vi "Actor Core.vi"(8 "error in":errorcluster, 11 "Bioreactor":refnum<class "Bioreactor.lvclass">) -> (0 "error out":errorcluster, 3 "Actor out":refnum<class "Actor.lvclass">)   [LabVIEW 2012, in "Bioreactor Actor.lvlib" / "Bioreactor.lvclass"]
doc: "This is Actor Core.vi, the main message handling loop for Actors. An actor usually just sits in this loop and processes messages as they arrive. Any error returned by the message Do.vi call will stop the loop, with error code 43 as the canonical signal to stop with no error sent to caller. Descendants may override that in Handle Error.vi."
uses:
  Bioreactor.lvclass
  <vilib>/ActorFramework/Actor/Actor.lvclass
  Bioreactor.lvclass/Bioreactor.ctl
  <vilib>/ActorFramework/Actor/Actor.lvclass/Actor.ctl
  <vilib>/ActorFramework/Message Enqueuer/Message Enqueuer.lvclass/Message Enqueuer.ctl
  <vilib>/ActorFramework/Message Enqueuer/Message Priority.ctl
  Read DVR.vi
  Write Loop Name.vi
  Write Graph History.vi
  Write Control Value.vi
  Write Control Graph.vi
  Write Process Setpoint.vi
  Write Process Value.vi
  Write Process Graph.vi
  Write VI Refnum.vi
  <vilib>/ActorFramework/Message Enqueuer/Init from Existing Queue.vi
  <vilib>/ActorFramework/Message Enqueuer/Enqueue.vi
  <vilib>/ActorFramework/Message Priority Queue/Priority Enqueue.vi
  <vilib>/ActorFramework/Message Enqueuer/Message Enqueuer.lvclass
  Bioreactor Messages/Read Setpoint Msg/Read Setpoint Msg.lvclass
  Bioreactor Messages/Read Output Msg/Read Output Msg.lvclass
  Bioreactor Messages/Read Value Msg/Read Value Msg.lvclass
  Bioreactor Messages/Update Indicators Msg/Update Indicators Msg.lvclass
  <vilib>/ActorFramework/Stop Msg/Stop Msg.lvclass
  Bioreactor Messages/Write Setpoint Msg/Write Setpoint Msg.lvclass
  Bioreactor Messages/Log Data Msg/Log Data Msg.lvclass
  Bioreactor Messages/Update Setpoint Msg/Update Setpoint Msg.lvclass
panel:
  in  "stop signal":bool
  out "Control Value":dbl=300.0
  in  "Graph History":dbl=300.0
  in  "Loop Name":u16(ring) caption="View"
  out "Control Graph":T1(graph) caption="Pump A"
  in  "Round Color Box 2":u32(colorbox)=16728642
  in  "Round Color Box":u32(colorbox)=483491
  in  "Process Setpoint":dbl=36.41913854673561
  out "Proccess Value":dbl=36.53012927910604
  out "Proccess Graph":T2(graph)
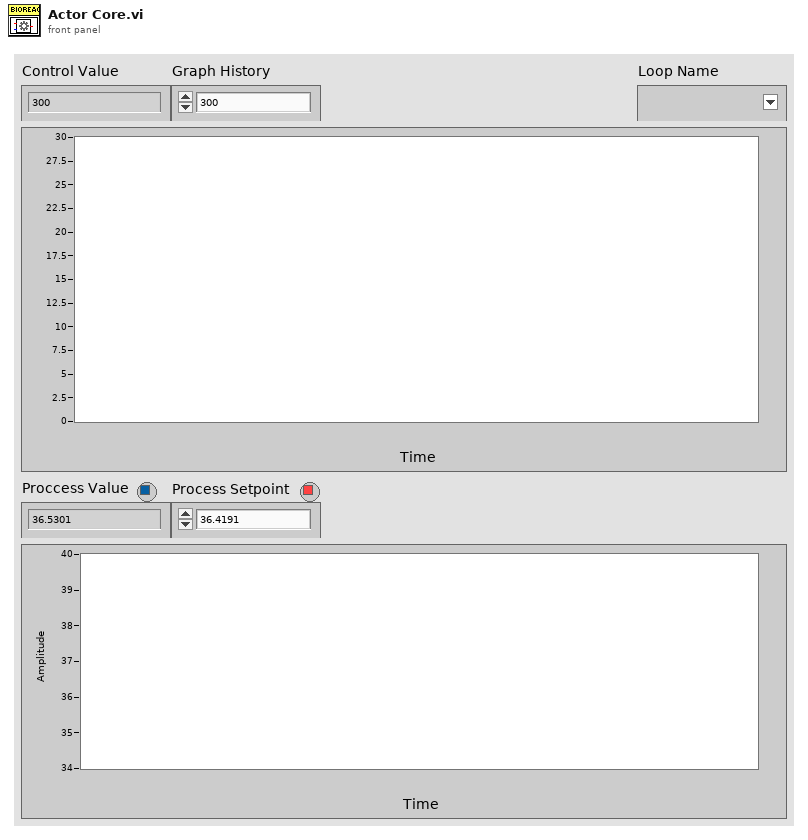
[diagram p1: front panel]
types:
  T1 = cluster{"output array":dbl[], "output array":dbl[]}
  T2 = cluster{"output array":dbl[], "output array":dbl[]}[]
  T3 = cluster{"Name":string, "Value":dbl, "Setpoint":dbl, "Output":dbl}[]
  T4 = typedef "Actor Framework.lvlib/Message Enqueuer.lvclass/Message Priority.ctl" = enum16{"Low", "Normal", "High"}
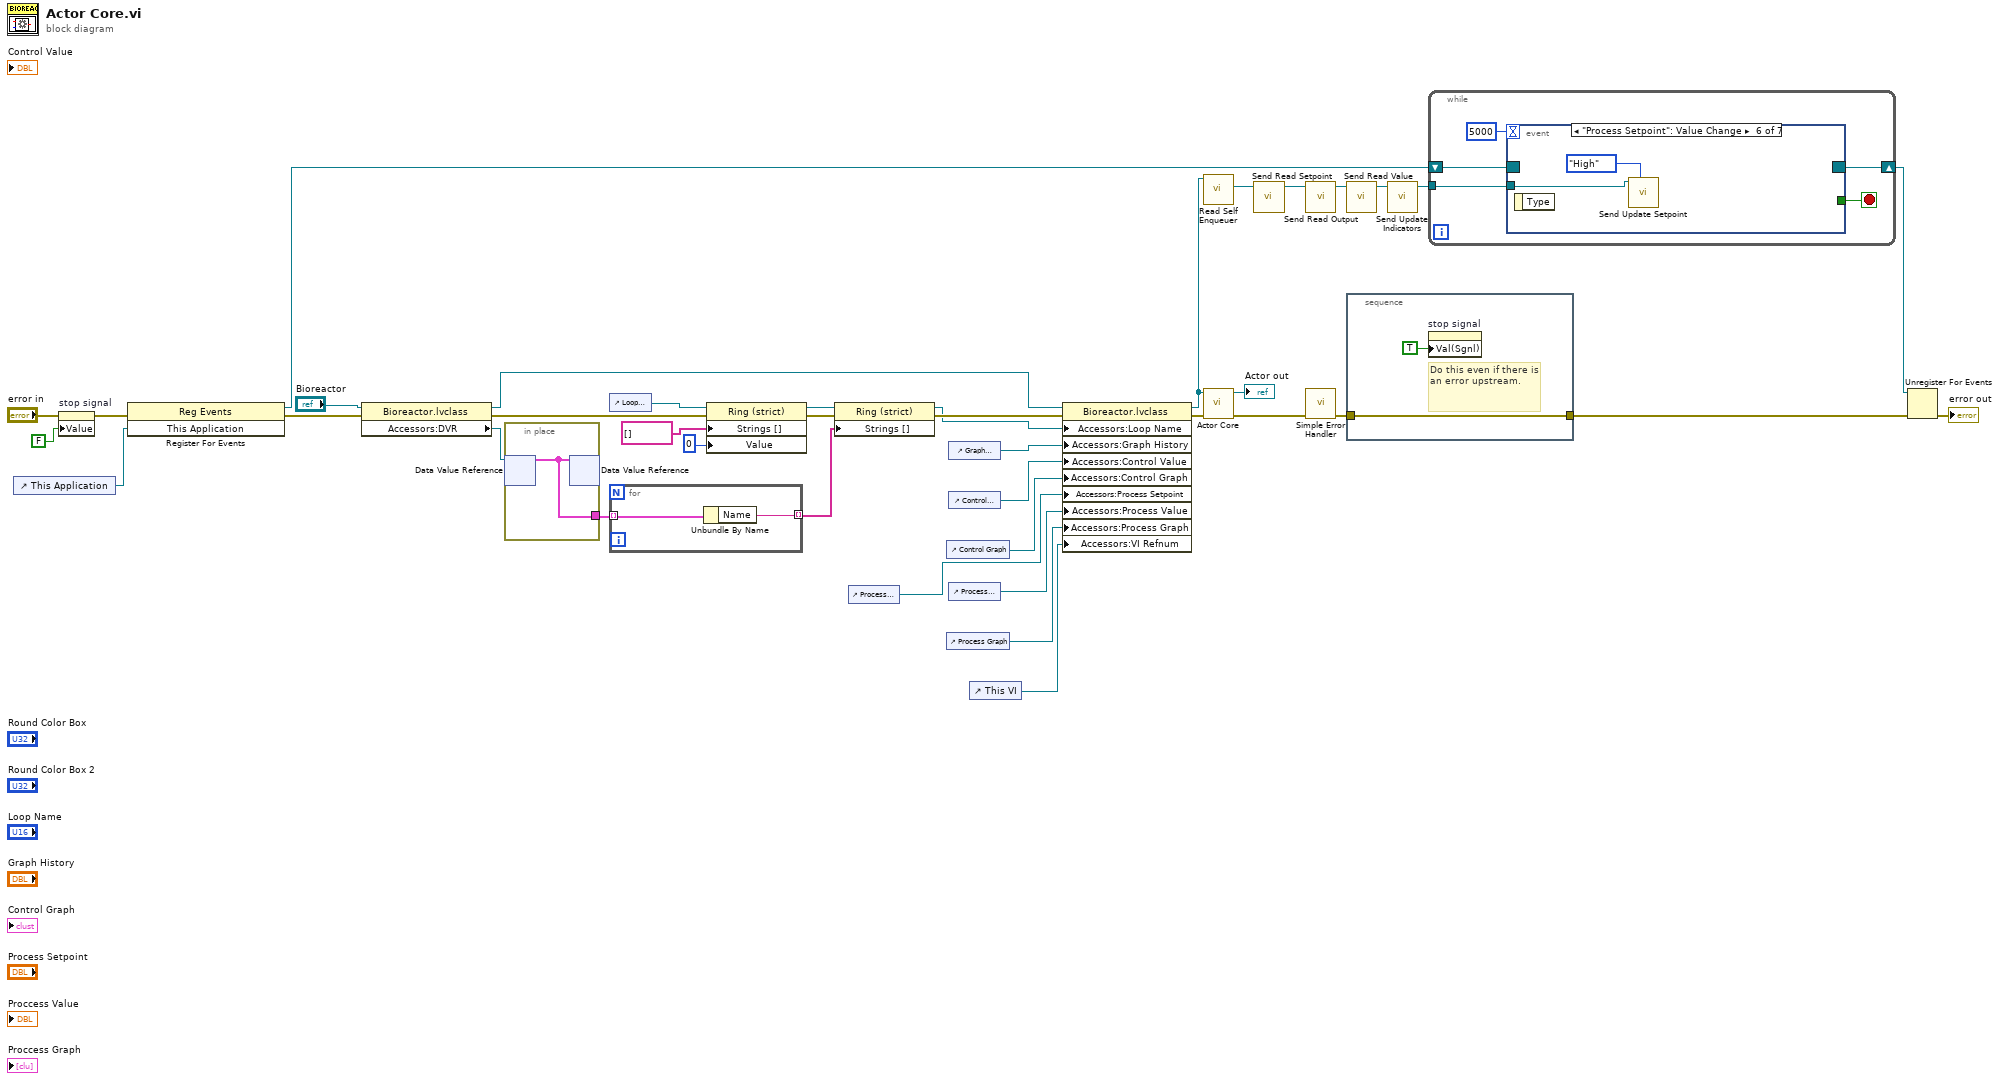
[diagram p0: block diagram]
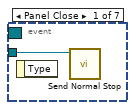
[diagram p2: hidden frame]
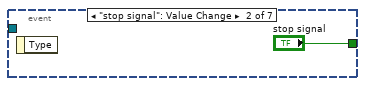
[diagram p3: hidden frame]
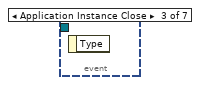
[diagram p4: hidden frame]
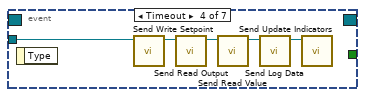
[diagram p5: hidden frame]
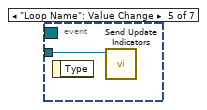
[diagram p6: hidden frame]
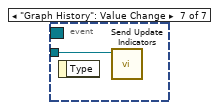
[diagram p7: hidden frame]
diagram:
  n1 = control-ref of="This Application"() -> (w32:refnum<vi>)
  n2 = property on="stop signal" class="Bool (strict)"(error in="error in", "Value"=FALSE ("stop")) -> (error out=w33:errorcluster)  [unwired: 1 in, 1 out]
  n3 = register-events(error in=w33, w32) -> (reference out=w36:refnum<event-registration>, error out=w19:errorcluster)  [unwired: 1 in]
  n4 = property class="Bioreactor.lvclass"(reference="Bioreactor", error in=w19) -> (reference out=w20:refnum<class "Bioreactor.lvclass">, error out=w3:errorcluster, "Accessors:DVR"=w18:refnum<data-value>)
  n5 = in-place {
    in-place-border: [w40] -> w17
    n6 = in-place-dvr #1(w18) -> (w40:T3)  [unwired: 1 out]
    n7 = in-place-dvr #1(w40) -> ()  [unwired: 2 out]
  }
  n8 = control-ref of="Loop Name"() -> (w5:refnum<vi>)
  n9 = for {
    tunnel: w17 -> [w42] mode=indexing
    tunnel: [w41] -> w15 mode=indexing
    n10 = Unbundle By Name(w42) -> ("Name"=w41:string)
  }
  n11 = property class="Ring (strict)"(reference=w5, error in=w3, "Strings []"=string[] [], "Value"=u16 0) -> (reference out=w4:refnum<vi>, error out=w2:errorcluster)
  n12 = property class="Ring (strict)"(reference=w4, error in=w2, "Strings []"=w15) -> (reference out=w14:refnum<vi>, error out=w16:errorcluster)
  n13 = control-ref of="Process Setpoint"() -> (w24:refnum<vi>)
  n14 = control-ref of="Control Graph"() -> (w25:refnum<vi>)
  n15 = control-ref of="Process Graph"() -> (w22:refnum<vi>)
  n16 = control-ref of="Graph History"() -> (w26:refnum<vi>)
  n17 = control-ref of="Control Value"() -> (w8:refnum<vi>)
  n18 = control-ref of="Process Value"() -> (w23:refnum<vi>)
  n19 = control-ref of="This VI"() -> (w13:refnum<vi>)
  n20 = property class="Bioreactor.lvclass"(reference=w20, error in=w16, "Accessors:Loop Name"=w14, "Accessors:Graph History"=w26, "Accessors:Control Value"=w8, "Accessors:Control Graph"=w25, "Accessors:Process Setpoint"=w24, "Accessors:Process Value"=w23, "Accessors:Process Graph"=w22, "Accessors:VI Refnum"=w13) -> (reference out=w30:refnum<class "Bioreactor.lvclass">, error out=w31:errorcluster)
  n21 = call <vilib>:"Read Self Enqueuer.vi"("Actor"=w30) -> ("Self Enqueuer"=w12:refnum<class "Message Enqueuer.lvclass">)  [unwired: 10 in]
  n22 = call-parent "Actor Core.vi"("error in"=w31, "Actor in"=w30) -> ("error out"=w38:errorcluster, "Actor out"=→"Actor out":refnum<class "Actor.lvclass">)  [unwired: 8 in]
  n23 = call "Send Read Setpoint.vi"("Message Enqueuer"=w12) -> ("Message Enqueuer out"=w7:refnum<class "Message Enqueuer.lvclass">)  [unwired: 9 in, 1 out]
  n24 = call "Send Read Output.vi"("Message Enqueuer"=w7) -> ("Message Enqueuer out"=w11:refnum<class "Message Enqueuer.lvclass">)  [unwired: 9 in, 1 out]
  n25 = call <vilib>:"Simple Error Handler.vi"("error in (no error)"=w38) -> ("error out"=w37:errorcluster)  [unwired: 4 in, 4 out]
  n26 = call "Send Read Value.vi"("Message Enqueuer"=w11) -> ("Message Enqueuer out"=w10:refnum<class "Message Enqueuer.lvclass">)  [unwired: 9 in, 1 out]
  n27 = stacked-sequence {
    tunnel: [w43] -> w34
    tunnel: w37 -> [w43]
    frame #0 {
      # "Do this even if there is an error upstream."
      n28 = property on="stop signal" class="Bool (strict)"("Val(Sgnl)"=TRUE ("stop")) -> ()  [unwired: 2 in, 2 out]
    }
  }
  n29 = call "Send Update Indicators.vi"("Message Enqueuer"=w10) -> ("Message Enqueuer out"=w9:refnum<class "Message Enqueuer.lvclass">)  [unwired: 9 in, 1 out]
  n30 = while {
    tunnel: w9 -> [w49]
    shift-right: [w46] -> w35
    shift-left: w36 -> [w47]
    stop <- w48 stop-if-true
    n31 = event shown="[5] \"Process Setpoint\": Value Change" {
      selector: w47 -> [_ _ _ _ _ _ _]
      dyn-events: [_ _ _ _ _ _ _] -> w46
      timeout: 5000 -> [_ _ _ _ _ _ _]
      tunnel: w49 -> [w50 _ _ w56 w57 w59 w60]
      tunnel: [_ "stop signal" _ _ _ _ _] -> w48
      event Panel Close {
        n32 = event-data() -> ()  [unwired: 1 in, 1 out]
        n33 = call <vilib>:"Send Normal Stop.vi"("Message Enqueuer"=w50) -> ()  [unwired: 10 in, 1 out]
      }
      event "stop signal": Value Change {
        n34 = event-data() -> ()  [unwired: 1 in, 1 out]
      }
      event Application Instance Close {
        n35 = event-data() -> ()  [unwired: 1 in, 1 out]
      }
      event Timeout {
        n36 = event-data() -> ()  [unwired: 1 in, 1 out]
        n37 = call "Send Write Setpoint.vi"("Message Enqueuer"=w56) -> ("Message Enqueuer out"=w55:refnum<class "Message Enqueuer.lvclass">)  [unwired: 9 in, 1 out]
        n38 = call "Send Read Output.vi"("Message Enqueuer"=w55) -> ("Message Enqueuer out"=w54:refnum<class "Message Enqueuer.lvclass">)  [unwired: 9 in, 1 out]
        n39 = call "Send Read Value.vi"("Message Enqueuer"=w54) -> ("Message Enqueuer out"=w53:refnum<class "Message Enqueuer.lvclass">)  [unwired: 9 in, 1 out]
        n40 = call "Send Log Data.vi"("Message Enqueuer"=w53) -> ("Message Enqueuer out"=w52:refnum<class "Message Enqueuer.lvclass">)  [unwired: 9 in, 1 out]
        n41 = call "Send Update Indicators.vi"("Message Enqueuer"=w52) -> ()  [unwired: 9 in, 2 out]
      }
      event "Loop Name": Value Change {
        n42 = event-data() -> ()  [unwired: 1 in, 1 out]
        n43 = call "Send Update Indicators.vi"("Message Enqueuer"=w57) -> ()  [unwired: 9 in, 2 out]
      }
      event "Process Setpoint": Value Change {
        n44 = event-data() -> ()  [unwired: 1 in, 1 out]
        n45 = call "Send Update Setpoint.vi"("Message Priority (Normal)"=Message_Priority."High", "Message Enqueuer"=w59) -> ()  [unwired: 8 in, 2 out]
      }
      event "Graph History": Value Change {
        n46 = event-data() -> ()  [unwired: 1 in, 1 out]
        n47 = call "Send Update Indicators.vi"("Message Enqueuer"=w60) -> ()  [unwired: 9 in, 2 out]
      }
    }
  }
  n48 = Unregister For Events(event registration refnum=w35, error in=w34) -> (error out=→"error out":errorcluster)
